vi "PP_assemble_tray_substract.vi"(8 "error in (no error)":errorcluster, 11 "DBlink":string="Driver={ODBC Driver 17 for SQL Server};Server=localhost\\SQLEXPRESS;Database=ZDX201;UID=labview;PWD=Dsa@54137926") -> (0 "error out":errorcluster, 2 "Result":T1)   [LabVIEW 2019]
uses:
  <vilib>/addons/database/Connection.llb/DB Tools Open Connec (String).vi
  <vilib>/addons/database/Connection.llb/Conn Execute.vi
  <vilib>/addons/database/Recordset.llb/Rec Destroy - Connection.vi
  <vilib>/addons/database/Recordset.llb/Rec Fetch Recordset Data (R).vi
  <vilib>/addons/database/_DB Variant To Data/Database Variant To Data.xnode
  <vilib>/addons/database/NI_Database_API.lvlib
panel:
  out "查詢結果":string="SELECT TOP (1000) [assemble_Tray]\n      ,[screw_A_Tray]\n      ,[screw_B_Tray]\n  FROM [ZDX201].[dbo].[preparation]"
  out "preparation":T2(array[cluster])
  out "減一指令":string
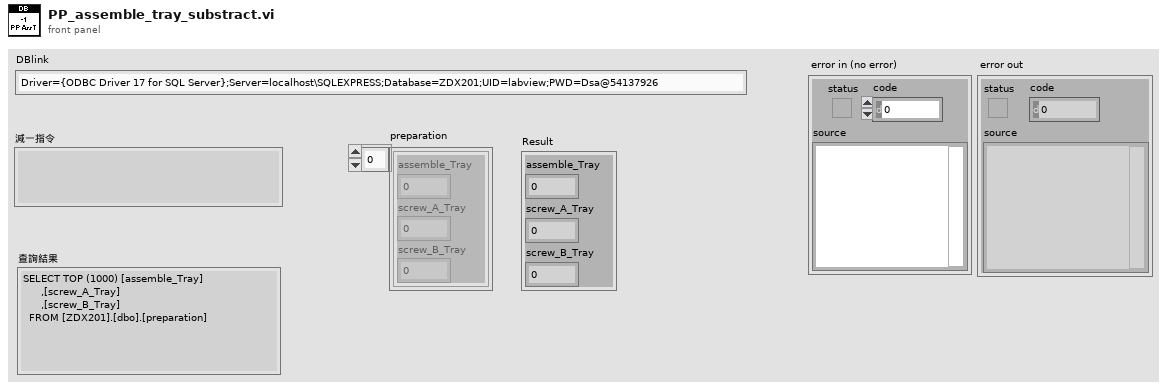
[diagram p1: front panel]
types:
  T1 = cluster{"assemble_Tray":i16, "screw_A_Tray":i16, "screw_B_Tray":i16}
  T2 = cluster{"assemble_Tray":i16, "screw_A_Tray":i16, "screw_B_Tray":i16}[]
  T3 = typedef "NI_Database_API.lvlib/Conn ObjectReference.ctl" = refnum<k1>
  T4 = typedef "NI_Database_API.lvlib/Rec ObjectReference.ctl" = refnum<k1>
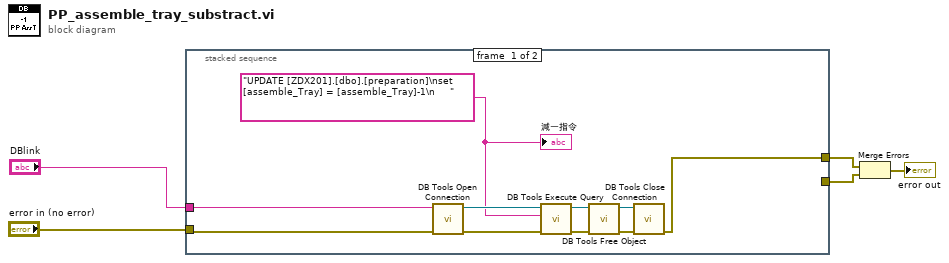
[diagram p0: block diagram]
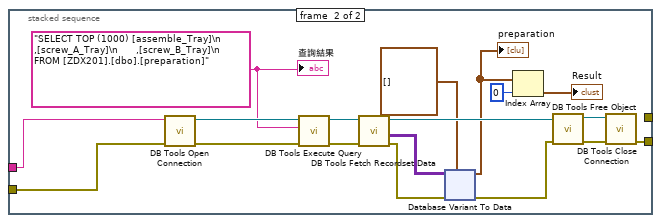
[diagram p2: hidden frame]
diagram:
  n1 = stacked-sequence {
    tunnel: "error in (no error)" -> [w8 w20]
    tunnel: "DBlink" -> [w7 w21]
    tunnel: [_ w19] -> w1
    tunnel: [w6 _] -> w2
    frame #0 {
      w9 = "UPDATE [ZDX201].[dbo].[preparation]\nset [assemble_Tray] = [assemble_Tray]-1\n     "
      n2 = call-poly <vilib>:"DB Tools Open Connection.vi"("error in (no error)"=w8, "connection information"=w7) -> ("error out"=w14:errorcluster, "connection reference"=w15:T3)  [unwired: 6 in]
      n3 = call-poly <vilib>:"DB Tools Execute Query.vi"("error in (no error)"=w14, "SQL query"=w9, "connection reference"=w15) -> ("error out"=w11:errorcluster, "recordset reference"=w12:T4)  [unwired: 5 in]
      n4 = call-poly <vilib>:"DB Tools Free Object.vi"("error in (no error)"=w11, "recordset reference"=w12) -> ("error out"=w10:errorcluster, "connection reference"=w13:T3)  [unwired: 8 in]
      n5 = call <vilib>:"DB Tools Close Connection.vi"("error in (no error)"=w10, "connection reference"=w13) -> ("error out"=w6:errorcluster)  [unwired: 5 in]
      "減一指令" <- w9
    }
    frame #1 {
      w23 = "SELECT TOP (1000) [assemble_Tray]\n      ,[screw_A_Tray]\n      ,[screw_B_Tray]\n  FROM [ZDX201].[dbo].[preparation]"
      n6 = call-poly <vilib>:"DB Tools Open Connection.vi"("error in (no error)"=w20, "connection information"=w21) -> ("error out"=w33:errorcluster, "connection reference"=w32:T3)  [unwired: 6 in]
      n7 = call-poly <vilib>:"DB Tools Execute Query.vi"("error in (no error)"=w33, "SQL query"=w23, "connection reference"=w32) -> ("error out"=w30:errorcluster, "recordset reference"=w31:T4)  [unwired: 5 in]
      n8 = call-poly <vilib>:"DB Tools Fetch Recordset Data.vi"("error in (no error)"=w30, "recordset reference"=w31) -> ("error out"=w25:errorcluster, "recordset data"=w24:variant[][], "recordset reference out"=w26:T4)  [unwired: 3 in]
      n9 = xnode "Database Variant To Data"("database variant"=w24, "error in (no error)"=w25, "type"=T2 [] ("Array")) -> ("data"=w18:T2, "error out"=w27:errorcluster)
      "preparation" <- w18
      n10 = Index Array(array=w18, index=0) -> (element=→"Result":T1)
      n11 = call-poly <vilib>:"DB Tools Free Object.vi"("error in (no error)"=w27, "recordset reference"=w26) -> ("error out"=w28:errorcluster, "connection reference"=w29:T3)  [unwired: 8 in]
      n12 = call <vilib>:"DB Tools Close Connection.vi"("error in (no error)"=w28, "connection reference"=w29) -> ("error out"=w19:errorcluster)  [unwired: 5 in]
      "查詢結果" <- w23
    }
  }
  n13 = Merge Errors(w2, w1) -> (→"error out":errorcluster)
